vi "DECLARE_IO.vi"(11 "TopLevelDiagram in":refnum<vi>) -> (1 "c_DECLARE_IO":string)   [LabVIEW 2017]
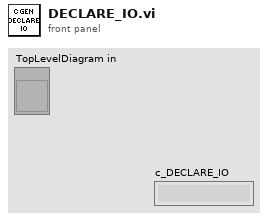
[diagram p1: front panel]
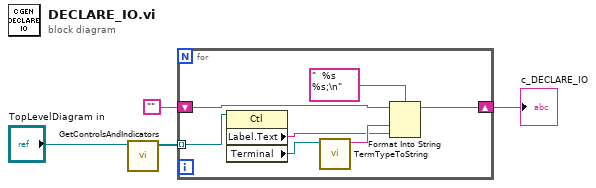
[diagram p0: block diagram]
diagram:
  n1 = call "GetControlsAndIndicators.vi"("TopLevelDiagram in"="TopLevelDiagram in") -> ("All ControlsTerminals"=w2:refnum<vi>[])  [unwired: 9 in, 1 out]
  n2 = for {
    tunnel: w2 -> [w11] mode=indexing
    shift-right: [w6] -> w3
    shift-left: "" -> [w5]
    n3 = property class="Ctl"(reference=w11) -> ("Label.Text"=w7:string, "Terminal"=w10:refnum<vi>)  [unwired: 1 in, 2 out]
    n4 = call "TermTypeToString.vi"("Terminal in"=w10) -> ("Name"=w8:string)  [unwired: 10 in]
    n5 = Format Into String(format string="  %s %s;\n", initial string=w5, w8, w7) -> (resulting string=w6:string)  [unwired: 1 in, 1 out]
  }
  "c_DECLARE_IO" <- w3
